vi "MGI Get Text Rect with Pad.vi"(2 "Text":string, 3 "Origin(0,0)":cluster{"horizontal":i16, "vertical":i16}, 4 "Font":T2) -> (0 "Width":i16, 1 "Rect":T1)   [LabVIEW 2020]
doc: "Measure text rect, then pad the width by 10% to correct for inaccuracies.\n\nAuthored by David A. Moore\nsupport@mooregoodideas.com\nwww.mooregoodideas.com\n\nCopyright (c) 2010, Moore Good Ideas, Inc.\n\nAll rights reserved.\n\nRedistribution and use in source and binary forms, with or without modification, are permitted provided that the following conditions are met:\n\n * Redistributions of source code must retain the above copyright notice, this list of conditions and the following disclaimer.\n * Redistributions in binary form must reproduce the above copyright notice, this list of conditions and the following disclaimer in the documentation and/or other materials provided with the distribution.\n * Neither the name of Moore Good Ideas, Inc. nor the names of its contributors may be used to endorse or promote products derived from this software without specific prior written permission.\n\nTHIS SOFTWARE IS PROVIDED BY THE COPYRIGHT HOLDERS AND CONTRIBUTORS \"AS IS\" AND ANY EXPRESS OR IMPLIED WARRANTIES, INCLUDING, BUT NOT LIMITED TO, THE IMPLIED WARRANTIES OF MERCHANTABILITY AND FITNESS FOR A PARTICULAR PURPOSE ARE DISCLAIMED. IN NO EVENT SHALL THE COPYRIGHT OWNER OR CONTRIBUTORS BE LIABLE FOR ANY DIRECT, INDIRECT, INCIDENTAL, SPECIAL, EXEMPLARY, OR CONSEQUENTIAL DAMAGES (INCLUDING, BUT NOT LIMITED TO, PROCUREMENT OF SUBSTITUTE GOODS OR SERVICES; LOSS OF USE, DATA, OR PROFITS; OR BUSINESS INTERRUPTION) HOWEVER CAUSED AND ON ANY THEORY OF LIABILITY, WHETHER IN CONTRACT, STRICT LIABILITY, OR TORT (INCLUDING NEGLIGENCE OR OTHERWISE) ARISING IN ANY WAY OUT OF THE USE OF THIS SOFTWARE, EVEN IF ADVISED OF THE POSSIBILITY OF SUCH DAMAGE."
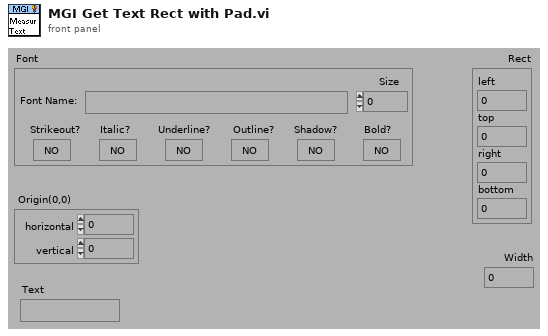
[diagram p1: front panel]
types:
  T1 = cluster{"left":i16, "top":i16, "right":i16, "bottom":i16}
  T2 = cluster{"Font Name:":string, "Size":i16, "Strikeout?":bool, "Italic?":bool, "Underline?":bool, "Outline?":bool, "Shadow?":bool, "Bold?":bool}
  T3 = enum16{"User-specified Font", "Application Font", "System Font", "Dialog Font"}
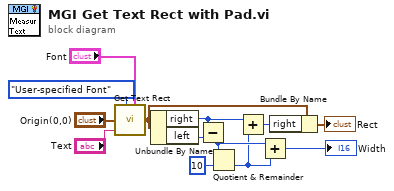
[diagram p0: block diagram]
diagram:
  n1 = call <vilib>:"Get Text Rect.vi"("desired font(Application)"=T3."User-specified Font" ("desired font(application)"), "origin(0,0)"="Origin(0,0)", "text"="Text", "[user-specified font]"="Font") -> ("rect"=w9:T1)  [unwired: 5 in]
  n2 = Unbundle By Name(w9) -> ("right"=w5:i16, "left"=w6:i16)
  n3 = Subtract(x=w5, y=w6) -> (x-y=w3:i16)
  n4 = Quotient & Remainder(x=w3, y=i16 10) -> (floor(x/y)=w2:i16)  [unwired: 1 out]
  n5 = Add(x=w5, y=w2) -> (x+y=w4:i16)
  n6 = Add(x=w3, y=w2) -> (x+y=→"Width":i16)
  n7 = Bundle By Name(cluster=w9, "right"=w4) -> (→"Rect":T1)
